vi "未命名 1.vi"() -> ()   [LabVIEW 2019]
panel:
  in  "XYGraph引用句柄":refnum<vi>
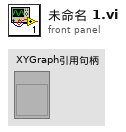
[diagram p1: front panel]
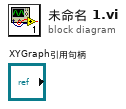
[diagram p0: block diagram]
diagram:
